vi "RTS Extract Contactor Settings.vi"(8 "Error In":errorcluster, 11 "Chamber 1 Socket":string[][](array[string])=[["System Date", "System Time", "Elapsed Time (sec)", "Elapsed Time (hrs)", "Voltage (V)", "RMS Current (Amps)", "Power (Watts)", "Watt Hours (Wh)", "Voltage Total Harmonic Distortion (%)", "Frequency (Hz)", "Apparent Power (VA)", "Power Factor", "TC 1", "TC 2", "TC 3", "TC 4", "TC 5", "TC 6", "TC 7", "TC 8", "TC 9", "TC 10", "TC 11", "TC 12", "TC 13", "TC 14", "TC 15", "TC 16", "TC 17", "TC 18", "TC 19", "TC 20", "TC 21", "TC 22", "TC 23", "TC 24", "TC 25", "TC 26", "TC 27", "TC 28", "TC 29", "TC 30", "AUX 1", "AUX 2", "CAL CL", "Room Setpoint Temperature", "Room Setpoint Humidity", "Room Temperature (°F)", "Room Humidity (%)", "Door Enable", "Room Setpoint Cool Temperature", "Room Setpoint Dehumidification Temperature", "Supply Temperature (°F)", "Cool Temperature (°F)", "Dehumidification Temperature (°F)", "Glycol Temperature (°F)", "Heat Rate (%)", "Steam Rate (%)", "Cool Rate (%)", "Dehumidification Rate (%)", "Room Status", "Room Dry P", "Room Dry I", "Room Humidity P", "Room Humidity I", "Room Heat P", "Room Heat I", "Room Cool Temperature P", "Room Cool Temperature I", "Room Dehumidification Temperature P", "Room Dehumidification Temperature I", "Voltage Setpoint 1", "60 Hz Power", "50 Hz Power", "120V Range", "240V Range", "Ground Line", "Ground Neutral", "Measure Ground Leakage Current", "Room OK", "S1 Freezer Relay", "S1 Cab Relay", "S1 Slide Relay", "Recording Data", "CVS Location", "Point Location"], ["01/23/2018", "12:12:48.917", "0.000000", "0.000000", "114.767563", "0.030115", "0.138006", "591.421923", "3.000000", "59.972565", "3.456177", "1.000000", "-1.540000", "-1.650000", "-0.660000", "327.670000", "327.670000", "327.670000", "327.670000", "327.670000", "327.670000", "327.670000", "38.080000", "36.100000", "35.660000", "327.670000", "327.670000", "327.670000", "327.670000", "327.670000", "327.670000", "327.670000", "327.670000", "327.670000", "327.670000", "70.140000", "327.670000", "327.670000", "70.270000", "327.670000", "32767.000000", "32767.000000", "0.000000", "0.000000", "1.988000", "70.000000", "35.000000", "70.040000", "38.130000", "1.000000", "55.000000", "48.000000", "66.790000", "55.000000", "47.890000", "0.000000", "38.260000", "0.000000", "31.060000", "9.080000", "0.000000", "200.000000", "15000.000000", "400.000000", "15000.000000", "1000.000000", "2000.000000", "500.000000", "6000.000000", "500.000000", "6000.000000", "115.000000", "1.000000", "0.000000", "1.000000", "0.000000", "0.000000", "1.000000", "0.000000", "1.000000", "0.000000", "0.000000", "0.000000", "FALSE", "", ""], ["System Date", "System Time", "Elapsed Time (sec)", "Elapsed Time (hrs)", "Voltage (V)", "RMS Current (Amps)", "Power (Watts)", "Watt Hours (Wh)", "Voltage Total Harmonic Distortion (%)", "Frequency (Hz)", "Apparent Power (VA)", "Power Factor", "TC 1", "TC 2", "TC 3", "TC 4", "TC 5", "TC 6", "TC 7", "TC 8", "TC 9", "TC 10", "TC 11", "TC 12", "TC 13", "TC 14", "TC 15", "TC 16", "TC 17", "TC 18", "TC 19", "TC 20", "TC 21", "TC 22", "TC 23", "TC 24", "TC 25", "TC 26", "TC 27", "TC 28", "TC 29", "TC 30", "AUX 1", "AUX 2", "CAL CL", "Room Setpoint Temperature", "Room Setpoint Humidity", "Room Temperature (°F)", "Room Humidity (%)", "Door Enable", "Room Setpoint Cool Temperature", "Room Setpoint Dehumidification Temperature", "Supply Temperature (°F)", "Cool Temperature (°F)", "Dehumidification Temperature (°F)", "Glycol Temperature (°F)", "Heat Rate (%)", "Steam Rate (%)", "Cool Rate (%)", "Dehumidification Rate (%)", "Room Status", "Room Dry P", "Room Dry I", "Room Humidity P", "Room Humidity I", "Room Heat P", "Room Heat I", "Room Cool Temperature P", "Room Cool Temperature I", "Room Dehumidification Temperature P", "Room Dehumidification Temperature I", "Voltage Setpoint 2", "60 Hz Power", "50 Hz Power", "120V Range", "240V Range", "Ground Line", "Ground Neutral", "Measure Ground Leakage Current", "Fault", "S2 Freezer Relay", "S2 Cab Relay", "S2 Slide Relay", "Recording Data", "CVS Location", "Point Location"], ["01/23/2018", "12:12:48.917", "0.000000", "0.000000", "115.354530", "0.030870", "0.137769", "25871.412688", "3.200000", "59.972309", "3.560970", "1.000000", "9.890000", "8.460000", "8.020000", "327.670000", "327.670000", "327.670000", "327.670000", "327.670000", "327.670000", "327.670000", "41.870000", "42.030000", "43.100000", "327.670000", "327.670000", "327.670000", "327.670000", "327.670000", "327.670000", "327.670000", "327.670000", "327.670000", "327.670000", "69.860000", "327.670000", "327.670000", "70.000000", "327.670000", "32767.000000", "32767.000000", "0.000000", "0.000000", "1.990000", "70.000000", "35.000000", "70.040000", "38.130000", "1.000000", "55.000000", "48.000000", "66.790000", "55.000000", "47.890000", "0.000000", "38.260000", "0.000000", "31.060000", "9.080000", "0.000000", "200.000000", "15000.000000", "400.000000", "15000.000000", "1000.000000", "2000.000000", "500.000000", "6000.000000", "500.000000", "6000.000000", "115.000000", "1.000000", "0.000000", "1.000000", "0.000000", "0.000000", "1.000000", "0.000000", "0.000000", "0.000000", "0.000000", "0.000000", "FALSE", "", ""], ["System Date", "System Time", "Elapsed Time (sec)", "Elapsed Time (hrs)", "Voltage (V)", "RMS Current (Amps)", "Power (Watts)", "Watt Hours (Wh)", "Voltage Total Harmonic Distortion (%)", "Frequency (Hz)", "Apparent Power (VA)", "Power Factor", "TC 1", "TC 2", "TC 3", "TC 4", "TC 5", "TC 6", "TC 7", "TC 8", "TC 9", "TC 10", "TC 11", "TC 12", "TC 13", "TC 14", "TC 15", "TC 16", "TC 17", "TC 18", "TC 19", "TC 20", "TC 21", "TC 22", "TC 23", "TC 24", "TC 25", "TC 26", "TC 27", "TC 28", "TC 29", "TC 30", "AUX 1", "AUX 2", "CAL CL", "Room Setpoint Temperature", "Room Setpoint Humidity", "Room Temperature (°F)", "Room Humidity (%)", "Door Enable", "Room Setpoint Cool Temperature", "Room Setpoint Dehumidification Temperature", "Supply Temperature (°F)", "Cool Temperature (°F)", "Dehumidification Temperature (°F)", "Glycol Temperature (°F)", "Heat Rate (%)", "Steam Rate (%)", "Cool Rate (%)", "Dehumidification Rate (%)", "Room Status", "Room Dry P", "Room Dry I", "Room Humidity P", "Room Humidity I", "Room Heat P", "Room Heat I", "Room Cool Temperature P", "Room Cool Temperature I", "Room Dehumidification Temperature P", "Room Dehumidification Temperature I", "Voltage Setpoint 3", "60 Hz Power", "50 Hz Power", "120V Range", "240V Range", "Ground Line", "Ground Neutral", "Measure Ground Leakage Current", "Room Heat", "S3 Freezer Relay", "S3 Cab Relay", "S3 Slide Relay", "Recording Data", "CVS Location", "Point Location"], ["01/23/2018", "12:12:48.918", "0.000000", "0.000000", "114.940773", "0.810396", "84.214592", "27582.388738", "3.300000", "59.972565", "93.147522", "0.904099", "9.420000", "7.550000", "6.540000", "327.670000", "327.670000", "327.670000", "327.670000", "327.670000", "327.670000", "327.670000", "40.710000", "40.580000", "40.990000", "327.670000", "327.670000", "327.670000", "327.670000", "327.670000", "327.670000", "327.670000", "327.670000", "327.670000", "327.670000", "69.920000", "327.670000", "327.670000", "70.770000", "327.670000", "32767.000000", "32767.000000", "0.000000", "0.000000", "1.963000", "70.000000", "35.000000", "70.040000", "38.130000", "1.000000", "55.000000", "48.000000", "66.790000", "55.000000", "47.890000", "0.000000", "38.260000", "0.000000", "31.060000", "9.080000", "0.000000", "200.000000", "15000.000000", "400.000000", "15000.000000", "1000.000000", "2000.000000", "500.000000", "6000.000000", "500.000000", "6000.000000", "115.000000", "1.000000", "0.000000", "1.000000", "0.000000", "0.000000", "1.000000", "0.000000", "1.000000", "0.000000", "0.000000", "0.000000", "FALSE", "", ""], ["System Date", "System Time", "Elapsed Time (sec)", "Elapsed Time (hrs)", "Voltage (V)", "RMS Current (Amps)", "Power (Watts)", "Watt Hours (Wh)", "Voltage Total Harmonic Distortion (%)", "Frequency (Hz)", "Apparent Power (VA)", "Power Factor", "TC 1", "TC 2", "TC 3", "TC 4", "TC 5", "TC 6", "TC 7", "TC 8", "TC 9", "TC 10", "TC 11", "TC 12", "TC 13", "TC 14", "TC 15", "TC 16", "TC 17", "TC 18", "TC 19", "TC 20", "TC 21", "TC 22", "TC 23", "TC 24", "TC 25", "TC 26", "TC 27", "TC 28", "TC 29", "TC 30", "AUX 1", "AUX 2", "CAL CL", "Room Setpoint Temperature", "Room Setpoint Humidity", "Room Temperature (°F)", "Room Humidity (%)", "Door Enable", "Room Setpoint Cool Temperature", "Room Setpoint Dehumidification Temperature", "Supply Temperature (°F)", "Cool Temperature (°F)", "Dehumidification Temperature (°F)", "Glycol Temperature (°F)", "Heat Rate (%)", "Steam Rate (%)", "Cool Rate (%)", "Dehumidification Rate (%)", "Room Status", "Room Dry P", "Room Dry I", "Room Humidity P", "Room Humidity I", "Room Heat P", "Room Heat I", "Room Cool Temperature P", "Room Cool Temperature I", "Room Dehumidification Temperature P", "Room Dehumidification Temperature I", "Voltage Setpoint 4", "60 Hz Power", "50 Hz Power", "120V Range", "240V Range", "Ground Line", "Ground Neutral", "Measure Ground Leakage Current", "Room Blower", "S4 Freezer Relay", "S4 Cab Relay", "S4 Slide Relay", "Recording Data", "CVS Location", "Point Location"], ["01/23/2018", "12:12:48.918", "0.000000", "0.000000", "115.354530", "0.030490", "0.136968", "26001.109791", "3.600000", "59.972996", "3.517112", "1.000000", "1.370000", "3.100000", "3.790000", "327.670000", "327.670000", "327.670000", "327.670000", "327.670000", "327.670000", "327.670000", "38.540000", "39.560000", "39.840000", "327.670000", "327.670000", "327.670000", "327.670000", "327.670000", "327.670000", "327.670000", "327.670000", "327.670000", "327.670000", "70.220000", "327.670000", "327.670000", "70.580000", "327.670000", "32767.000000", "32767.000000", "0.000000", "0.000000", "2.005000", "70.000000", "35.000000", "70.040000", "38.130000", "1.000000", "55.000000", "48.000000", "66.790000", "55.000000", "47.890000", "0.000000", "38.260000", "0.000000", "31.060000", "9.080000", "0.000000", "200.000000", "15000.000000", "400.000000", "15000.000000", "1000.000000", "2000.000000", "500.000000", "6000.000000", "500.000000", "6000.000000", "115.000000", "1.000000", "0.000000", "1.000000", "0.000000", "0.000000", "1.000000", "0.000000", "1.000000", "0.000000", "0.000000", "0.000000", "FALSE", "", ""], ["System Date", "System Time", "Elapsed Time (sec)", "Elapsed Time (hrs)", "Voltage (V)", "RMS Current (Amps)", "Power (Watts)", "Watt Hours (Wh)", "Voltage Total Harmonic Distortion (%)", "Frequency (Hz)", "Apparent Power (VA)", "Power Factor", "TC 1", "TC 2", "TC 3", "TC 4", "TC 5", "TC 6", "TC 7", "TC 8", "TC 9", "TC 10", "TC 11", "TC 12", "TC 13", "TC 14", "TC 15", "TC 16", "TC 17", "TC 18", "TC 19", "TC 20", "TC 21", "TC 22", "TC 23", "TC 24", "TC 25", "TC 26", "TC 27", "TC 28", "TC 29", "TC 30", "AUX 1", "AUX 2", "CAL CL", "Room Setpoint Temperature", "Room Setpoint Humidity", "Room Temperature (°F)", "Room Humidity (%)", "Door Enable", "Room Setpoint Cool Temperature", "Room Setpoint Dehumidification Temperature", "Supply Temperature (°F)", "Cool Temperature (°F)", "Dehumidification Temperature (°F)", "Glycol Temperature (°F)", "Heat Rate (%)", "Steam Rate (%)", "Cool Rate (%)", "Dehumidification Rate (%)", "Room Status", "Room Dry P", "Room Dry I", "Room Humidity P", "Room Humidity I", "Room Heat P", "Room Heat I", "Room Cool Temperature P", "Room Cool Temperature I", "Room Dehumidification Temperature P", "Room Dehumidification Temperature I", "Voltage Setpoint 5", "60 Hz Power", "50 Hz Power", "120V Range", "240V Range", "Ground Line", "Ground Neutral", "Measure Ground Leakage Current", "Spare", "S5 Freezer Relay", "S5 Cab Relay", "S5 Slide Relay", "Recording Data", "CVS Location", "Point Location"], ["01/23/2018", "12:12:48.918", "0.000000", "0.000000", "114.979256", "0.000000", "0.000000", "0.000000", "3.100000", "59.973503", "0.000000", "1.000000", "327.670000", "327.670000", "70.220000", "327.670000", "327.670000", "327.670000", "327.670000", "327.670000", "327.670000", "327.670000", "70.440000", "70.160000", "70.160000", "327.670000", "327.670000", "327.670000", "327.670000", "327.670000", "327.670000", "327.670000", "327.670000", "327.670000", "327.670000", "69.860000", "327.670000", "327.670000", "327.670000", "327.670000", "32767.000000", "32767.000000", "0.000000", "0.000000", "1.999000", "70.000000", "35.000000", "70.040000", "38.130000", "1.000000", "55.000000", "48.000000", "66.790000", "55.000000", "47.890000", "0.000000", "38.260000", "0.000000", "31.060000", "9.080000", "0.000000", "200.000000", "15000.000000", "400.000000", "15000.000000", "1000.000000", "2000.000000", "500.000000", "6000.000000", "500.000000", "6000.000000", "115.000000", "1.000000", "0.000000", "1.000000", "0.000000", "0.000000", "1.000000", "0.000000", "0.000000", "0.000000", "0.000000", "0.000000", "FALSE", "", ""], ["System Date", "System Time", "Elapsed Time (sec)", "Elapsed Time (hrs)", "Voltage (V)", "RMS Current (Amps)", "Power (Watts)", "Watt Hours (Wh)", "Voltage Total Harmonic Distortion (%)", "Frequency (Hz)", "Apparent Power (VA)", "Power Factor", "TC 1", "TC 2", "TC 3", "TC 4", "TC 5", "TC 6", "TC 7", "TC 8", "TC 9", "TC 10", "TC 11", "TC 12", "TC 13", "TC 14", "TC 15", "TC 16", "TC 17", "TC 18", "TC 19", "TC 20", "TC 21", "TC 22", "TC 23", "TC 24", "TC 25", "TC 26", "TC 27", "TC 28", "TC 29", "TC 30", "AUX 1", "AUX 2", "CAL CL", "Room Setpoint Temperature", "Room Setpoint Humidity", "Room Temperature (°F)", "Room Humidity (%)", "Door Enable", "Room Setpoint Cool Temperature", "Room Setpoint Dehumidification Temperature", "Supply Temperature (°F)", "Cool Temperature (°F)", "Dehumidification Temperature (°F)", "Glycol Temperature (°F)", "Heat Rate (%)", "Steam Rate (%)", "Cool Rate (%)", "Dehumidification Rate (%)", "Room Status", "Room Dry P", "Room Dry I", "Room Humidity P", "Room Humidity I", "Room Heat P", "Room Heat I", "Room Cool Temperature P", "Room Cool Temperature I", "Room Dehumidification Temperature P", "Room Dehumidification Temperature I", "Voltage Setpoint 6", "60 Hz Power", "50 Hz Power", "120V Range", "240V Range", "Ground Line", "Ground Neutral", "Measure Ground Leakage Current", "Room Pump", "S6 Freezer Relay", "S6 Cab Relay", "S6 Slide Relay", "Recording Data", "CVS Location", "Point Location"], ["01/23/2018", "12:12:48.918", "0.000000", "0.000000", "114.738701", "0.000000", "0.000000", "0.000000", "3.500000", "59.973148", "0.000000", "1.000000", "327.670000", "327.670000", "327.670000", "327.670000", "327.670000", "327.670000", "327.670000", "327.670000", "327.670000", "327.670000", "327.670000", "327.670000", "327.670000", "327.670000", "327.670000", "327.670000", "327.670000", "327.670000", "327.670000", "327.670000", "327.670000", "327.670000", "327.670000", "327.670000", "327.670000", "327.670000", "327.670000", "327.670000", "32767.000000", "32767.000000", "0.000000", "0.000000", "1.995000", "70.000000", "35.000000", "70.040000", "38.130000", "1.000000", "55.000000", "48.000000", "66.790000", "55.000000", "47.890000", "0.000000", "38.260000", "0.000000", "31.060000", "9.080000", "0.000000", "200.000000", "15000.000000", "400.000000", "15000.000000", "1000.000000", "2000.000000", "500.000000", "6000.000000", "500.000000", "6000.000000", "115.000000", "1.000000", "0.000000", "1.000000", "0.000000", "0.000000", "1.000000", "0.000000", "1.000000", "0.000000", "0.000000", "0.000000", "FALSE", "", ""], ["System Date", "System Time", "Elapsed Time (sec)", "Elapsed Time (hrs)", "Voltage (V)", "RMS Current (Amps)", "Power (Watts)", "Watt Hours (Wh)", "Voltage Total Harmonic Distortion (%)", "Frequency (Hz)", "Apparent Power (VA)", "Power Factor", "TC 1", "TC 2", "TC 3", "TC 4", "TC 5", "TC 6", "TC 7", "TC 8", "TC 9", "TC 10", "TC 11", "TC 12", "TC 13", "TC 14", "TC 15", "TC 16", "TC 17", "TC 18", "TC 19", "TC 20", "TC 21", "TC 22", "TC 23", "TC 24", "TC 25", "TC 26", "TC 27", "TC 28", "TC 29", "TC 30", "AUX 1", "AUX 2", "CAL CL", "Room Setpoint Temperature", "Room Setpoint Humidity", "Room Temperature (°F)", "Room Humidity (%)", "Door Enable", "Room Setpoint Cool Temperature", "Room Setpoint Dehumidification Temperature", "Supply Temperature (°F)", "Cool Temperature (°F)", "Dehumidification Temperature (°F)", "Glycol Temperature (°F)", "Heat Rate (%)", "Steam Rate (%)", "Cool Rate (%)", "Dehumidification Rate (%)", "Room Status", "Room Dry P", "Room Dry I", "Room Humidity P", "Room Humidity I", "Room Heat P", "Room Heat I", "Room Cool Temperature P", "Room Cool Temperature I", "Room Dehumidification Temperature P", "Room Dehumidification Temperature I", "Voltage Setpoint 7", "60 Hz Power", "50 Hz Power", "120V Range", "240V Range", "Ground Line", "Ground Neutral", "Measure Ground Leakage Current", "Spare", "S7 Freezer Relay", "S7 Cab Relay", "S7 Slide Relay", "Recording Data", "CVS Location", "Point Location"], ["01/23/2018", "12:12:48.919", "0.000000", "0.000000", "114.960014", "0.000000", "0.000000", "0.000000", "3.500000", "59.972225", "0.000000", "1.000000", "70.580000", "70.630000", "70.630000", "327.670000", "327.670000", "327.670000", "327.670000", "327.670000", "327.670000", "327.670000", "327.670000", "70.440000", "70.490000", "327.670000", "327.670000", "327.670000", "327.670000", "327.670000", "327.670000", "327.670000", "327.670000", "327.670000", "327.670000", "327.670000", "327.670000", "327.670000", "327.670000", "327.670000", "32767.000000", "32767.000000", "0.000000", "0.000000", "2.003000", "70.000000", "35.000000", "70.040000", "38.130000", "1.000000", "55.000000", "48.000000", "66.790000", "55.000000", "47.890000", "0.000000", "38.260000", "0.000000", "31.060000", "9.080000", "0.000000", "200.000000", "15000.000000", "400.000000", "15000.000000", "1000.000000", "2000.000000", "500.000000", "6000.000000", "500.000000", "6000.000000", "115.000000", "1.000000", "0.000000", "1.000000", "0.000000", "0.000000", "1.000000", "0.000000", "0.000000", "0.000000", "0.000000", "0.000000", "FALSE", "", ""], ["System Date", "System Time", "Elapsed Time (sec)", "Elapsed Time (hrs)", "Voltage (V)", "RMS Current (Amps)", "Power (Watts)", "Watt Hours (Wh)", "Voltage Total Harmonic Distortion (%)", "Frequency (Hz)", "Apparent Power (VA)", "Power Factor", "TC 1", "TC 2", "TC 3", "TC 4", "TC 5", "TC 6", "TC 7", "TC 8", "TC 9", "TC 10", "TC 11", "TC 12", "TC 13", "TC 14", "TC 15", "TC 16", "TC 17", "TC 18", "TC 19", "TC 20", "TC 21", "TC 22", "TC 23", "TC 24", "TC 25", "TC 26", "TC 27", "TC 28", "TC 29", "TC 30", "AUX 1", "AUX 2", "CAL CL", "Room Setpoint Temperature", "Room Setpoint Humidity", "Room Temperature (°F)", "Room Humidity (%)", "Door Enable", "Room Setpoint Cool Temperature", "Room Setpoint Dehumidification Temperature", "Supply Temperature (°F)", "Cool Temperature (°F)", "Dehumidification Temperature (°F)", "Glycol Temperature (°F)", "Heat Rate (%)", "Steam Rate (%)", "Cool Rate (%)", "Dehumidification Rate (%)", "Room Status", "Room Dry P", "Room Dry I", "Room Humidity P", "Room Humidity I", "Room Heat P", "Room Heat I", "Room Cool Temperature P", "Room Cool Temperature I", "Room Dehumidification Temperature P", "Room Dehumidification Temperature I", "Voltage Setpoint 8", "60 Hz Power", "50 Hz Power", "120V Range", "240V Range", "Ground Line", "Ground Neutral", "Measure Ground Leakage Current", "Spare", "S8 Freezer Relay", "S8 Cab Relay", "S8 Slide Relay", "Recording Data", "CVS Location", "Point Location"], ["01/23/2018", "12:12:48.919", "0.000000", "0.000000", "115.190956", "0.000000", "0.000000", "0.000000", "3.500000", "59.972149", "0.000000", "1.000000", "70.580000", "70.410000", "70.490000", "327.670000", "327.670000", "327.670000", "327.670000", "327.670000", "327.670000", "327.670000", "70.630000", "70.360000", "70.300000", "327.670000", "327.670000", "327.670000", "327.670000", "327.670000", "327.670000", "327.670000", "327.670000", "327.670000", "327.670000", "327.670000", "327.670000", "327.670000", "327.670000", "327.670000", "32767.000000", "32767.000000", "0.000000", "0.000000", "1.954000", "70.000000", "35.000000", "70.040000", "38.130000", "1.000000", "55.000000", "48.000000", "66.790000", "55.000000", "47.890000", "0.000000", "38.260000", "0.000000", "31.060000", "9.080000", "0.000000", "200.000000", "15000.000000", "400.000000", "15000.000000", "1000.000000", "2000.000000", "500.000000", "6000.000000", "500.000000", "6000.000000", "115.000000", "1.000000", "0.000000", "1.000000", "0.000000", "0.000000", "1.000000", "0.000000", "0.000000", "0.000000", "0.000000", "0.000000", "FALSE", "", ""]]) -> (0 "Error Out":errorcluster, 2 "Current Contactor Settings":T1, 3 "Current Door Output Relays Status":T3)   [LabVIEW 2020]
uses:
  Drivers/WAGO 750-881/Type Definitions/Wago Door Relays.ctl
  Drivers/WAGO 750-881/Type Definitions/Wago Contactor Settings.ctl
  Drivers/WAGO 750-881/Type Definitions/Wago Ground Leakage.ctl
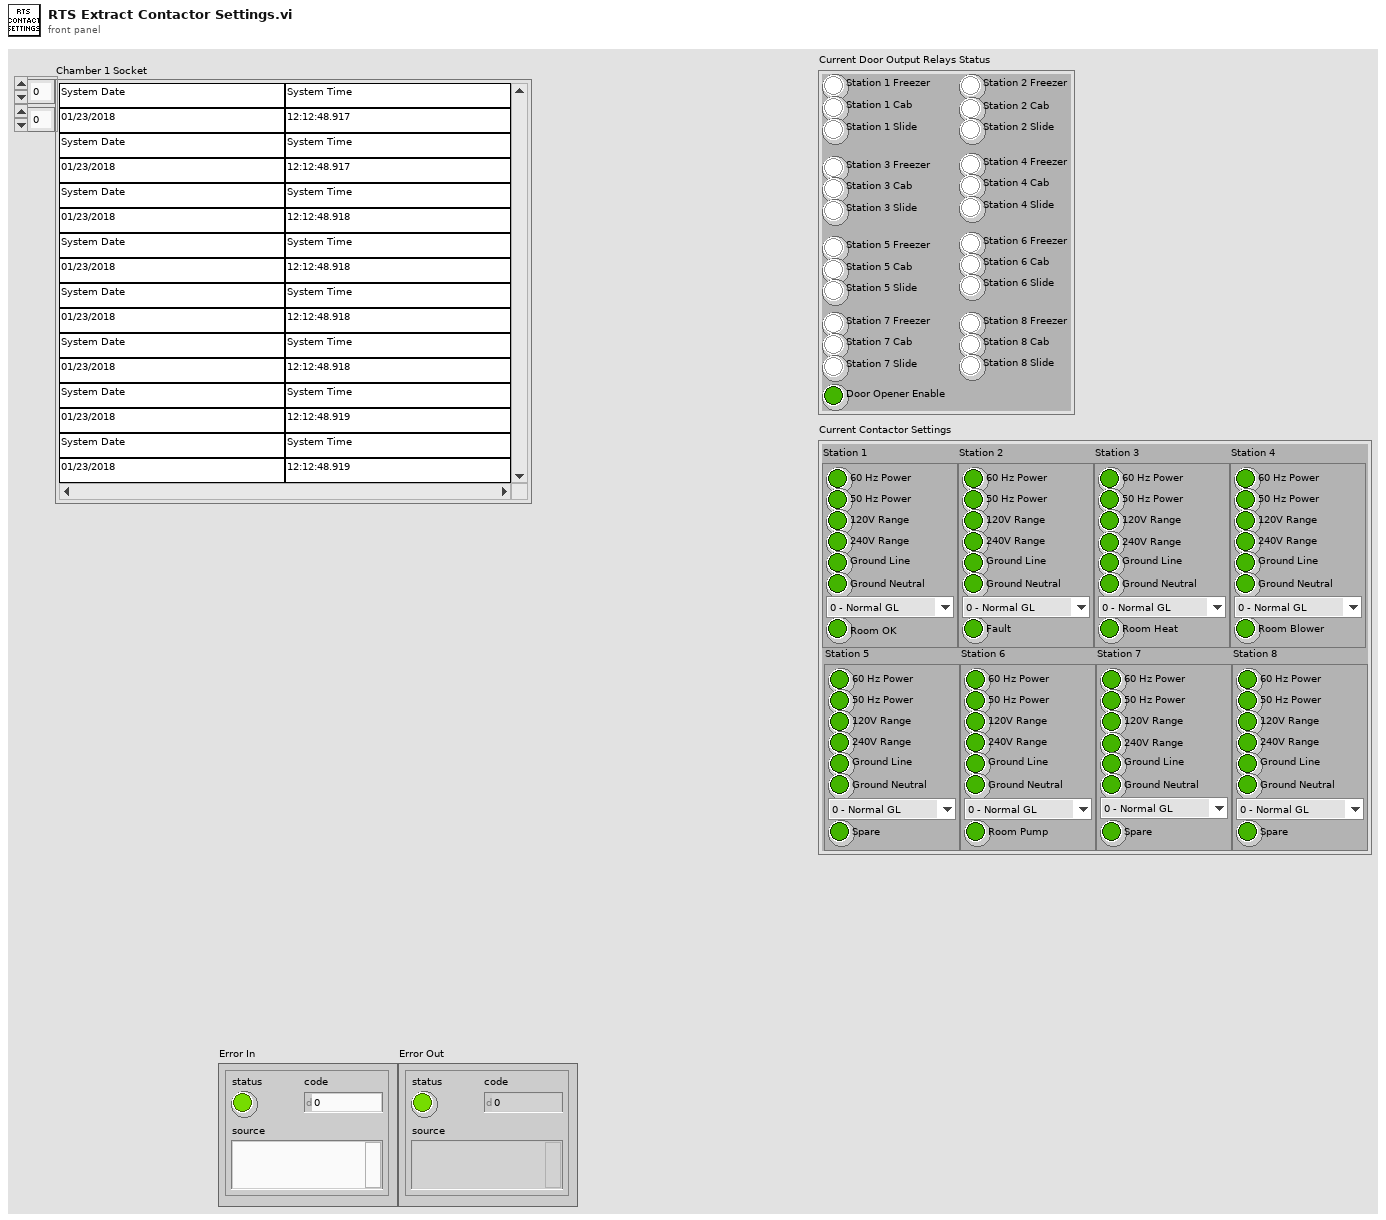
[diagram p1: front panel]
types:
  T1 = typedef "Wago Contactor Settings.ctl" = cluster{"Station 1":cluster{"60 Hz Power":bool, "50 Hz Power":bool, "120V Range":bool, "240V Range":bool, "Ground Line":bool, "Ground Neutral":bool, "Room OK":bool, "Ground Leakage":T2}, "Station 2":cluster{"60 Hz Power":bool, "50 Hz Power":bool, "120V Range":bool, "240V Range":bool, "Ground Line":bool, "Ground Neutral":bool, "Fault":bool, "Ground Leakage":T2}, "Station 3":cluster{"60 Hz Power":bool, "50 Hz Power":bool, "120V Range":bool, "240V Range":bool, "Ground Line":bool, "Ground Neutral":bool, "Room Heat":bool, "Ground Leakage":T2}, "Station 4":cluster{"60 Hz Power":bool, "50 Hz Power":bool, "120V Range":bool, "240V Range":bool, "Ground Line":bool, "Ground Neutral":bool, "Room Blower":bool, "Ground Leakage":T2}, "Station 5":cluster{"60 Hz Power":bool, "50 Hz Power":bool, "120V Range":bool, "240V Range":bool, "Ground Line":bool, "Ground Neutral":bool, "Spare":bool, "Ground Leakage":T2}, "Station 6":cluster{"60 Hz Power":bool, "50 Hz Power":bool, "120V Range":bool, "240V Range":bool, "Ground Line":bool, "Ground Neutral":bool, "Room Pump":bool, "Ground Leakage":T2}, "Station 7":cluster{"60 Hz Power":bool, "50 Hz Power":bool, "120V Range":bool, "240V Range":bool, "Ground Line":bool, "Ground Neutral":bool, "Spare":bool, "Ground Leakage":T2}, "Station 8":cluster{"60 Hz Power":bool, "50 Hz Power":bool, "120V Range":bool, "240V Range":bool, "Ground Line":bool, "Ground Neutral":bool, "Spare":bool, "Ground Leakage":T2}}
  T2 = typedef "Wago Ground Leakage.ctl" = enum16{"0 - Normal GL", "1 - Measure GL"}
  T3 = typedef "Wago Door Relays.ctl" = cluster{"Station 1 Freezer":bool, "Station 1 Cab":bool, "Station 1 Slide":bool, "Station 2 Freezer":bool, "Station 2 Cab":bool, "Station 2 Slide":bool, "Station 3 Freezer":bool, "Station 3 Cab":bool, "Station 3 Slide":bool, "Station 4 Freezer":bool, "Station 4 Cab":bool, "Station 4 Slide":bool, "Station 5 Freezer":bool, "Station 5 Cab":bool, "Station 5 Slide":bool, "Station 6 Freezer":bool, "Station 6 Cab":bool, "Station 6 Slide":bool, "Station 7 Freezer":bool, "Station 7 Cab":bool, "Station 7 Slide":bool, "Station 8 Freezer":bool, "Station 8 Cab":bool, "Station 8 Slide":bool, "Door Opener Enable":bool}
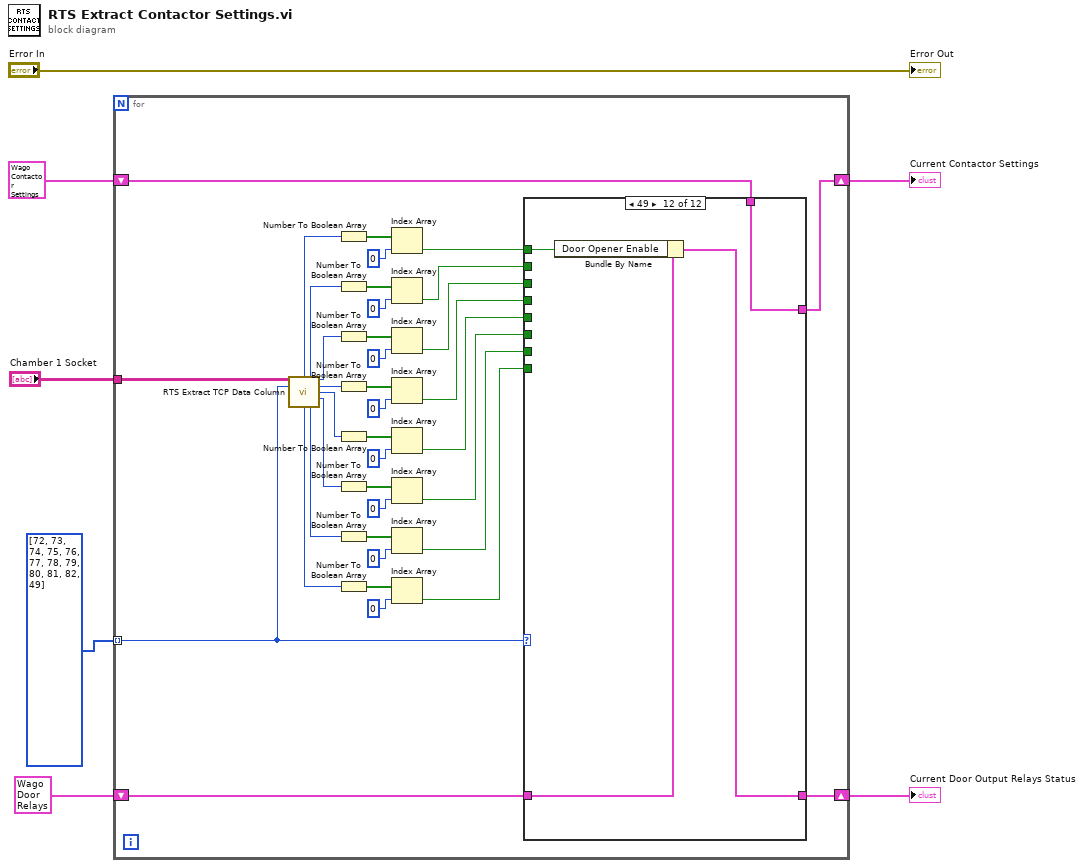
[diagram p0: block diagram]
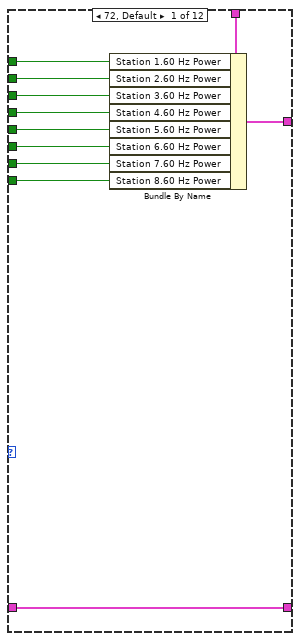
[diagram p2: hidden frame]
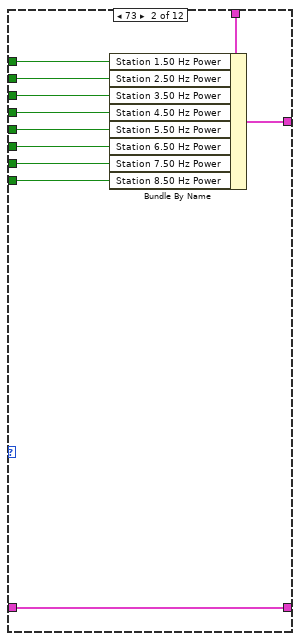
[diagram p3: hidden frame]
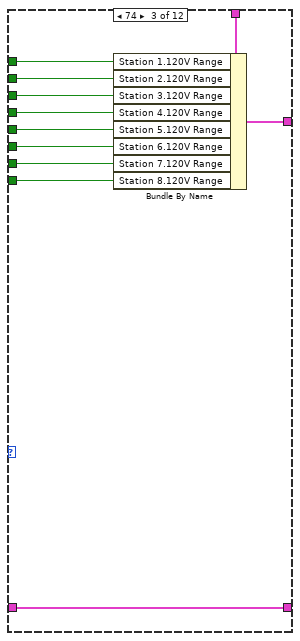
[diagram p4: hidden frame]
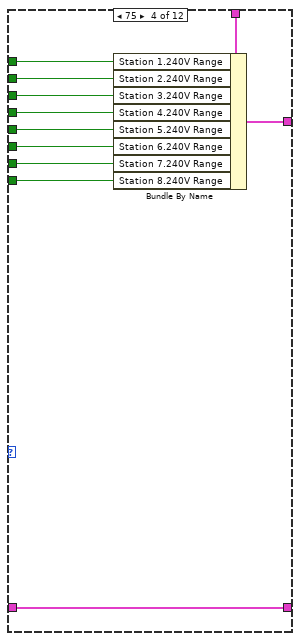
[diagram p5: hidden frame]
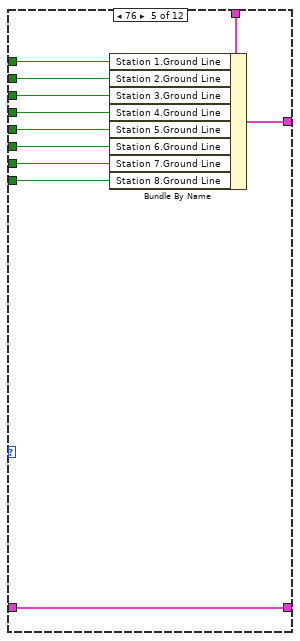
[diagram p6: hidden frame]
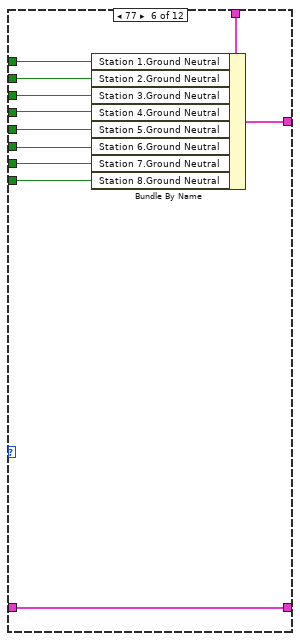
[diagram p7: hidden frame]
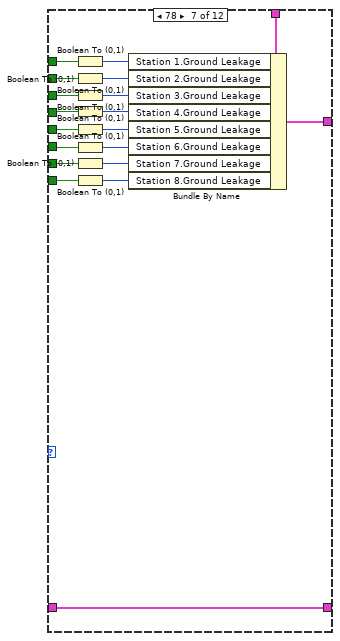
[diagram p8: hidden frame]
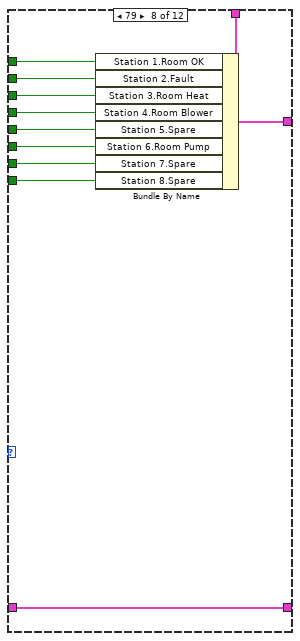
[diagram p9: hidden frame]
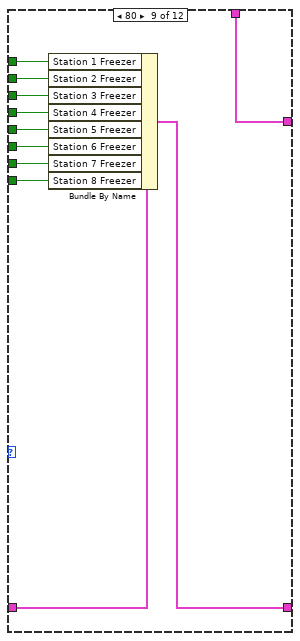
[diagram p10: hidden frame]
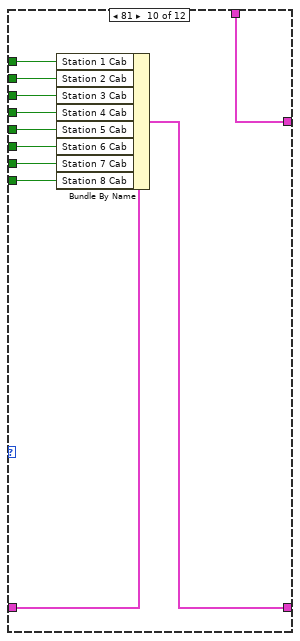
[diagram p11: hidden frame]
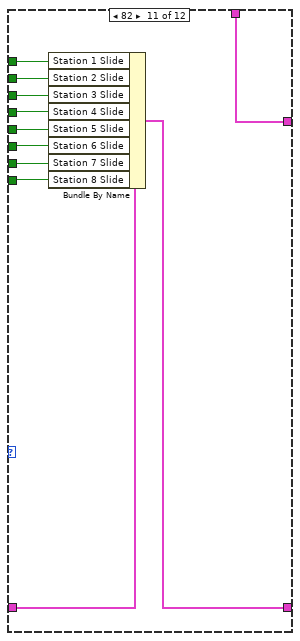
[diagram p12: hidden frame]
diagram:
  n1 = for {
    tunnel: "Chamber 1 Socket" -> [w13]
    shift-right: [w12] -> w4
    shift-left: T1 {"Station 1"={"60 Hz Power"=FALSE, "50 Hz Power"=FALSE, "120V Range"=FALSE, "240V Range"=FALSE, "Ground Line"=FALSE, "Ground Neutral"=FALSE, "Room OK"=FALSE, "Ground Leakage"=enum."0 - Normal GL"}, "Station 2"={"60 Hz Power"=FALSE, "50 Hz Power"=FALSE, "120V Range"=FALSE, "240V Range"=FALSE, "Ground Line"=FALSE, "Ground Neutral"=FALSE, "Fault"=FALSE, "Ground Leakage"=enum."0 - Normal GL"}, "Station 3"={"60 Hz Power"=FALSE, "50 Hz Power"=FALSE, "120V Range"=FALSE, "240V Range"=FALSE, "Ground Line"=FALSE, "Ground Neutral"=FALSE, "Room Heat"=FALSE, "Ground Leakage"=enum."0 - Normal GL"}, "Station 4"={"60 Hz Power"=FALSE, "50 Hz Power"=FALSE, "120V Range"=FALSE, "240V Range"=FALSE, "Ground Line"=FALSE, "Ground Neutral"=FALSE, "Room Blower"=FALSE, "Ground Leakage"=enum."0 - Normal GL"}, "Station 5"={"60 Hz Power"=FALSE, "50 Hz Power"=FALSE, "120V Range"=FALSE, "240V Range"=FALSE, "Ground Line"=FALSE, "Ground Neutral"=FALSE, "Spare"=FALSE, "Ground Leakage"=enum."0 - Normal GL"}, "Station 6"={"60 Hz Power"=FALSE, "50 Hz Power"=FALSE, "120V Range"=FALSE, "240V Range"=FALSE, "Ground Line"=FALSE, "Ground Neutral"=FALSE, "Room Pump"=FALSE, "Ground Leakage"=enum."0 - Normal GL"}, "Station 7"={"60 Hz Power"=FALSE, "50 Hz Power"=FALSE, "120V Range"=FALSE, "240V Range"=FALSE, "Ground Line"=FALSE, "Ground Neutral"=FALSE, "Spare"=FALSE, "Ground Leakage"=enum."0 - Normal GL"}, "Station 8"={"60 Hz Power"=FALSE, "50 Hz Power"=FALSE, "120V Range"=FALSE, "240V Range"=FALSE, "Ground Line"=FALSE, "Ground Neutral"=FALSE, "Spare"=FALSE, "Ground Leakage"=enum."0 - Normal GL"}} ("Current Contactor Settings") -> [w11]
    tunnel: i32[] [72, 73, 74, 75, 76, 77, 78, 79, 80, 81, 82, 49] -> [w10] mode=indexing
    shift-right: [w8] -> w1
    shift-left: T3 {"Station 1 Freezer"=FALSE, "Station 1 Cab"=FALSE, "Station 1 Slide"=FALSE, "Station 2 Freezer"=FALSE, "Station 2 Cab"=FALSE, "Station 2 Slide"=FALSE, "Station 3 Freezer"=FALSE, "Station 3 Cab"=FALSE, "Station 3 Slide"=FALSE, "Station 4 Freezer"=FALSE, "Station 4 Cab"=FALSE, "Station 4 Slide"=FALSE, "Station 5 Freezer"=FALSE, "Station 5 Cab"=FALSE, "Station 5 Slide"=FALSE, "Station 6 Freezer"=FALSE, "Station 6 Cab"=FALSE, "Station 6 Slide"=FALSE, "Station 7 Freezer"=FALSE, "Station 7 Cab"=FALSE, "Station 7 Slide"=FALSE, "Station 8 Freezer"=FALSE, "Station 8 Cab"=FALSE, "Station 8 Slide"=FALSE, "Door Opener Enable"=FALSE} ("Current Door Output Relays Status") -> [w9]
    n2 = call "RTS Extract TCP Data Column.vi"("Chamber 1 Socket"=w13, "Extract Column"=w10) -> ("Station 1"=w44:i32, "Station 2"=w39:i32, "Station 3"=w36:i32, "Station 4"=w34:i32, "Station 5"=w31:i32, "Station 6"=w27:i32, "Station 8"=w21:i32, "Station 7"=w24:i32)  [unwired: 5 in, 1 out]
    n3 = Number To Boolean Array(number=w44) -> (Boolean array=w43:bool[])
    n4 = Number To Boolean Array(number=w39) -> (Boolean array=w41:bool[])
    n5 = Number To Boolean Array(number=w36) -> (Boolean array=w37:bool[])
    n6 = Number To Boolean Array(number=w34) -> (Boolean array=w33:bool[])
    n7 = Number To Boolean Array(number=w31) -> (Boolean array=w30:bool[])
    n8 = Number To Boolean Array(number=w27) -> (Boolean array=w29:bool[])
    n9 = Number To Boolean Array(number=w24) -> (Boolean array=w25:bool[])
    n10 = Number To Boolean Array(number=w21) -> (Boolean array=w23:bool[])
    n11 = Index Array(array=w43, index=0) -> (element=w42:bool)
    n12 = Index Array(array=w41, index=0) -> (element=w20:bool)
    n13 = Index Array(array=w37, index=0) -> (element=w19:bool)
    n14 = Index Array(array=w33, index=0) -> (element=w18:bool)
    n15 = Index Array(array=w30, index=0) -> (element=w17:bool)
    n16 = Index Array(array=w29, index=0) -> (element=w16:bool)
    n17 = Index Array(array=w25, index=0) -> (element=w15:bool)
    n18 = Index Array(array=w23, index=0) -> (element=w14:bool)
    n19 = case shown="49" w10 {
      tunnel: w42 -> [w56 w65 w76 w87 w98 w109 w120 w139 w149 w161 w171 w175]
      tunnel: w20 -> [w55 w64 w75 w86 w97 w108 w119 w138 w148 w160 w170 _]
      tunnel: w19 -> [w54 w63 w74 w85 w96 w107 w118 w137 w147 w159 w169 _]
      tunnel: w18 -> [w53 w62 w73 w84 w95 w106 w117 w136 w146 w158 w168 _]
      tunnel: w17 -> [w52 w61 w72 w83 w94 w105 w116 w135 w145 w157 w167 _]
      tunnel: w16 -> [w51 w60 w71 w82 w93 w104 w115 w134 w144 w156 w166 _]
      tunnel: w15 -> [w50 w59 w70 w81 w92 w103 w114 w133 w143 w155 w165 _]
      tunnel: w14 -> [w49 w58 w69 w80 w91 w102 w113 w132 w142 w154 w164 _]
      tunnel: [w48 w66 w77 w88 w99 w110 w121 w140 w150 w153 w172 w178] -> w12
      tunnel: w11 -> [w47 w67 w78 w89 w100 w111 w122 w141 w150 w153 w172 w178]
      tunnel: w9 -> [w46 w57 w68 w79 w90 w101 w112 w131 w152 w163 w174 w177]
      tunnel: [w46 w57 w68 w79 w90 w101 w112 w131 w151 w162 w173 w176] -> w8
      frame 72, Default {
        n20 = Bundle By Name(cluster=w47, "Station 1.60 Hz Power"=w56, "Station 2.60 Hz Power"=w55, "Station 3.60 Hz Power"=w54, "Station 4.60 Hz Power"=w53, "Station 5.60 Hz Power"=w52, "Station 6.60 Hz Power"=w51, "Station 7.60 Hz Power"=w50, "Station 8.60 Hz Power"=w49) -> (w48:T1)
      }
      frame 73 {
        n21 = Bundle By Name(cluster=w67, "Station 1.50 Hz Power"=w65, "Station 2.50 Hz Power"=w64, "Station 3.50 Hz Power"=w63, "Station 4.50 Hz Power"=w62, "Station 5.50 Hz Power"=w61, "Station 6.50 Hz Power"=w60, "Station 7.50 Hz Power"=w59, "Station 8.50 Hz Power"=w58) -> (w66:T1)
      }
      frame 74 {
        n22 = Bundle By Name(cluster=w78, "Station 1.120V Range"=w76, "Station 2.120V Range"=w75, "Station 3.120V Range"=w74, "Station 4.120V Range"=w73, "Station 5.120V Range"=w72, "Station 6.120V Range"=w71, "Station 7.120V Range"=w70, "Station 8.120V Range"=w69) -> (w77:T1)
      }
      frame 75 {
        n23 = Bundle By Name(cluster=w89, "Station 1.240V Range"=w87, "Station 2.240V Range"=w86, "Station 3.240V Range"=w85, "Station 4.240V Range"=w84, "Station 5.240V Range"=w83, "Station 6.240V Range"=w82, "Station 7.240V Range"=w81, "Station 8.240V Range"=w80) -> (w88:T1)
      }
      frame 76 {
        n24 = Bundle By Name(cluster=w100, "Station 1.Ground Line"=w98, "Station 2.Ground Line"=w97, "Station 3.Ground Line"=w96, "Station 4.Ground Line"=w95, "Station 5.Ground Line"=w94, "Station 6.Ground Line"=w93, "Station 7.Ground Line"=w92, "Station 8.Ground Line"=w91) -> (w99:T1)
      }
      frame 77 {
        n25 = Bundle By Name(cluster=w111, "Station 1.Ground Neutral"=w109, "Station 2.Ground Neutral"=w108, "Station 3.Ground Neutral"=w107, "Station 4.Ground Neutral"=w106, "Station 5.Ground Neutral"=w105, "Station 6.Ground Neutral"=w104, "Station 7.Ground Neutral"=w103, "Station 8.Ground Neutral"=w102) -> (w110:T1)
      }
      frame 78 {
        n26 = Boolean To (0,1)(Boolean=w120) -> (0, 1=w130:i16)
        n27 = Boolean To (0,1)(Boolean=w119) -> (0, 1=w129:i16)
        n28 = Boolean To (0,1)(Boolean=w118) -> (0, 1=w128:i16)
        n29 = Boolean To (0,1)(Boolean=w117) -> (0, 1=w127:i16)
        n30 = Boolean To (0,1)(Boolean=w116) -> (0, 1=w126:i16)
        n31 = Boolean To (0,1)(Boolean=w115) -> (0, 1=w125:i16)
        n32 = Boolean To (0,1)(Boolean=w114) -> (0, 1=w124:i16)
        n33 = Boolean To (0,1)(Boolean=w113) -> (0, 1=w123:i16)
        n34 = Bundle By Name(cluster=w122, "Station 1.Ground Leakage"=w130, "Station 2.Ground Leakage"=w129, "Station 3.Ground Leakage"=w128, "Station 4.Ground Leakage"=w127, "Station 5.Ground Leakage"=w126, "Station 6.Ground Leakage"=w125, "Station 7.Ground Leakage"=w124, "Station 8.Ground Leakage"=w123) -> (w121:T1)
      }
      frame 79 {
        n35 = Bundle By Name(cluster=w141, "Station 1.Room OK"=w139, "Station 2.Fault"=w138, "Station 3.Room Heat"=w137, "Station 4.Room Blower"=w136, "Station 5.Spare"=w135, "Station 6.Room Pump"=w134, "Station 7.Spare"=w133, "Station 8.Spare"=w132) -> (w140:T1)
      }
      frame 80 {
        n36 = Bundle By Name(cluster=w152, "Station 1 Freezer"=w149, "Station 2 Freezer"=w148, "Station 3 Freezer"=w147, "Station 4 Freezer"=w146, "Station 5 Freezer"=w145, "Station 6 Freezer"=w144, "Station 7 Freezer"=w143, "Station 8 Freezer"=w142) -> (w151:T3)
      }
      frame 81 {
        n37 = Bundle By Name(cluster=w163, "Station 1 Cab"=w161, "Station 2 Cab"=w160, "Station 3 Cab"=w159, "Station 4 Cab"=w158, "Station 5 Cab"=w157, "Station 6 Cab"=w156, "Station 7 Cab"=w155, "Station 8 Cab"=w154) -> (w162:T3)
      }
      frame 82 {
        n38 = Bundle By Name(cluster=w174, "Station 1 Slide"=w171, "Station 2 Slide"=w170, "Station 3 Slide"=w169, "Station 4 Slide"=w168, "Station 5 Slide"=w167, "Station 6 Slide"=w166, "Station 7 Slide"=w165, "Station 8 Slide"=w164) -> (w173:T3)
      }
      frame 49 {
        n39 = Bundle By Name(cluster=w177, "Door Opener Enable"=w175) -> (w176:T3)
      }
    }
  }
  "Current Door Output Relays Status" <- w1
  "Current Contactor Settings" <- w4
  "Error Out" <- "Error In"
